vi "Read Attributes.vi"(11 "UserInfo Msg":refnum<class "UserInfo Msg.lvclass">) -> (2 "Payload":T3)   [LabVIEW 2019, in "UserManagement.lvlib" / "UserInfo Msg.lvclass"]
uses:
  UserInfo Msg.lvclass
  UserManagement/UserInfo.ctl
  UserManagement/Permission.ctl
  UserInfo Msg.lvclass/UserInfo Msg.ctl
  UserManagement/UserManagement.lvclass
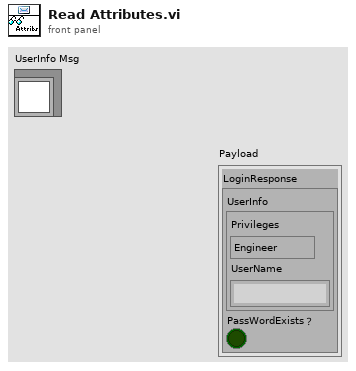
[diagram p1: front panel]
types:
  T1 = typedef "UserManagement.lvlib/UserManagement.lvclass/UserInfo.ctl" = cluster{"Privileges":T2, "UserName":string}
  T2 = typedef "UserManagement.lvlib/UserManagement.lvclass/Permission.ctl" = enum16{"Engineer", "Technical", "Operator"}
  T3 = cluster{"LoginResponse":cluster{"UserInfo":T1, "PassWordExists？":bool}}
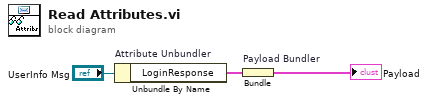
[diagram p0: block diagram]
diagram:
  n1 = Unbundle By Name "Attribute Unbundler"("UserInfo Msg") -> ("LoginResponse"=w1:cluster{"UserInfo":T1, "PassWordExists？":bool})
  n2 = Bundle "Payload Bundler"("LoginResponse"=w1) -> (→"Payload":T3)  [unwired: 1 in]
